vi "benchmark.vi"() -> ()   [LabVIEW 2017]
panel:
  out "x/y 4":dbl
  out "x/y 3":dbl
  out "x/y 2":dbl
  out "x/y":dbl
  out "write tagcontainer":dbl=3.782166481018067e-05 caption="write" format="%#_6f"
  out "read tagcontainer":dbl=3.934283256530761e-05 caption="read" format="%#_6f"
  out "write datacontainer":dbl=7.281229972839357e-07 caption="write" format="%#_6f"
  out "read datacontainer":dbl=1.454608345031738e-06 caption="read" format="%#_6f"
  out "write xnode":dbl=2.78111743927002e-05 caption="write" format="%#_6f"
  out "read xnode":dbl=2.8434400558471685e-05 caption="read" format="%#_6f"
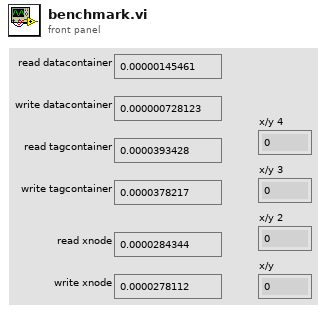
[diagram p1: front panel]
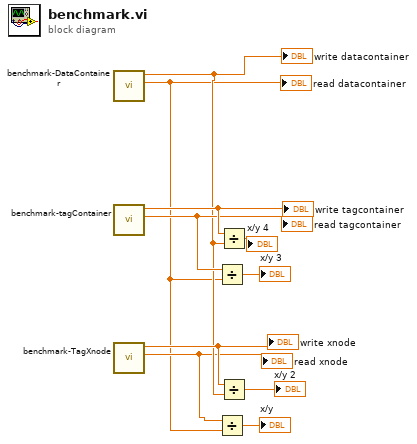
[diagram p0: block diagram]
diagram:
  n1 = call "benchmark-DataContainer.vi"() -> ("read"=w5:dbl, "write"=w7:dbl)  [unwired: 10 in]
  "read datacontainer" <- w5
  "write datacontainer" <- w7
  n2 = call "benchmark-tagContainer.vi"() -> ("read"=w9:dbl, "write"=w10:dbl)  [unwired: 10 in]
  "read tagcontainer" <- w9
  "write tagcontainer" <- w10
  n3 = call "benchmark-TagXnode.vi"() -> ("read"=w6:dbl, "write"=w8:dbl)  [unwired: 10 in]
  "read xnode" <- w6
  "write xnode" <- w8
  n4 = Divide(x=w9, y=w5) -> (x/y=→"x/y 3":dbl)
  n5 = Divide(x=w6, y=w5) -> (x/y=→"x/y":dbl)
  n6 = Divide(x=w10, y=w7) -> (x/y=→"x/y 4":dbl)
  n7 = Divide(x=w8, y=w7) -> (x/y=→"x/y 2":dbl)
